vi "PB Uninit.vi"(2 "Container State":T1, 3 "Display State":T2={"Window Handle"=refnum, "Maximum"=100, "State Change Action"=enum."Method - Initialize", "Running"=FALSE, "Visable Items"={"Label"=TRUE, "Caption"=FALSE}, "Value"=100, "Show Progress Bar"=FALSE}) -> ()   [LabVIEW 2011, in "Taskbar Progress Bar.xctl"]
uses:
  Taskbar Progress Bar.xctl
  PB State.ctl
  TypeDefs/Dispaly State Change Methods.ctl
  <vilib>/_xctls/Container State.ctl
  <vilib>/_xctls/XControlSupport.lvlib
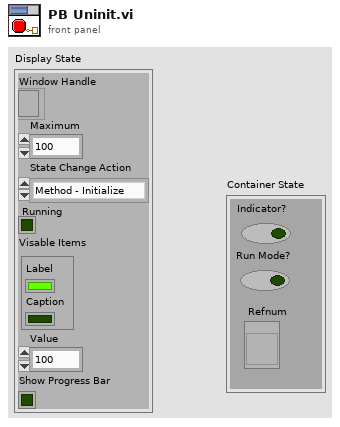
[diagram p1: front panel]
types:
  T1 = typedef "XControlSupport.lvlib/Container State.ctl" = cluster{"Indicator?":bool, "Run Mode?":bool, " Refnum":refnum<vi>}
  T2 = typedef "Taskbar Progress Bar.xctl/PB State.ctl" = cluster{"Window Handle":refnum<k24>, "Maximum":u64, "State Change Action":T3, "Running":bool, "Visable Items":cluster{"Label":bool, "Caption":bool}, "Value":u64, "Show Progress Bar":bool}
  T3 = typedef "Taskbar Progress Bar.xctl/Dispaly State Change Methods.ctl" = enum16{"No Action", "Created", "Method - Initialize", "Method - Increment", "Method - Pause", "Method - Error", "Method - Finish", "Property - Show Progress Bar"}
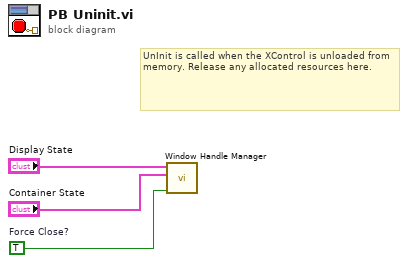
[diagram p0: block diagram]
diagram:
  w1 = TRUE  # Force Close?
  # "UnInit is called when the XControl is unloaded from memory. Release any allocated resources here."
  n1 = call "Window Handle Manager.vi"("Force Close?"=w1, "Container State"="Container State", "Display State in"="Display State") -> ()  [unwired: 8 in, 1 out]
